vi "DT_Triangle Manager_Add Boundary.vi"(5 "point 2":i32, 6 "CCW? [T]":bool=TRUE, 7 "triangle 2":i32, 8 "point 1":i32, 9 "triangle 1":i32, 10 "apex point":i32, 11 "Triangles In":i32[][](array[numeric])) -> (0 "new triangle 2":i32, 1 "new triangle 1":i32, 2 "triangle":i32, 3 "Triangles Out":i32[][](array[numeric]))   [LabVIEW 2017, in "NI_AAL_Geometry.lvlib"]
uses:
  <vilib>/Analysis/NI_AAL_Geometry.lvlib
  <vilib>/Analysis/geometry.llb/DT_Triangle Manager_Get Global Point Index.vi
  <vilib>/Analysis/geometry.llb/DT_Triangle Manager_Get Oppo Point_in Ghost.vi
  <vilib>/Analysis/geometry.llb/DT_Triangle Manager_Get Oppo Point.vi
  <vilib>/Analysis/geometry.llb/DT_Triangle Manager_Default Ghost Index.vi
  <vilib>/Analysis/geometry.llb/DT_Triangle Manager_Get Ghost Point.vi
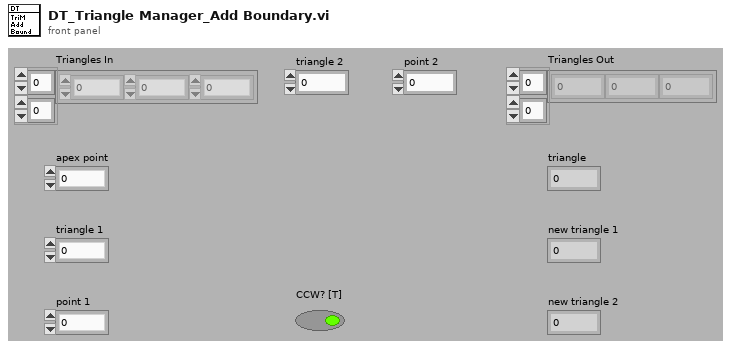
[diagram p1: front panel]
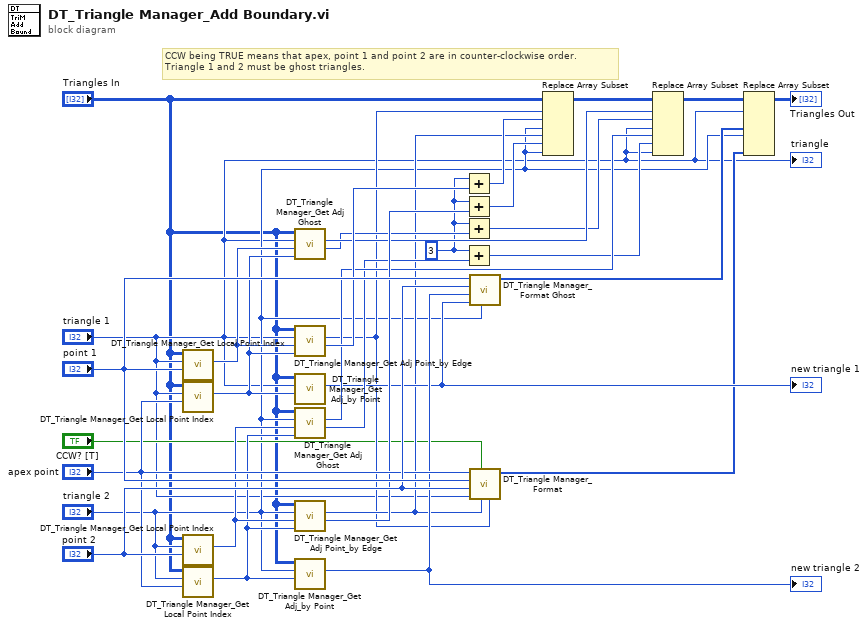
[diagram p0: block diagram]
diagram:
  w11 = 3 ("y")
  # "CCW being TRUE means that apex, point 1 and point 2 are in counter-clockwise order.\nTriangle 1 and 2 must be ghost triangles."
  n1 = call <vilib>:"DT_Triangle Manager_Get Local Point Index.vi"("global idx"="point 1", "triangle"="triangle 1", "Triangles"="Triangles In") -> ("local idx"=w23:i32)  [unwired: 8 out]
  n2 = call <vilib>:"DT_Triangle Manager_Get Local Point Index.vi"("global idx"="apex point", "triangle"="triangle 1", "Triangles"="Triangles In") -> ("local idx"=w22:i32)  [unwired: 8 out]
  n3 = call <vilib>:"DT_Triangle Manager_Get Local Point Index.vi"("global idx"="point 2", "triangle"="triangle 2", "Triangles"="Triangles In") -> ("local idx"=w18:i32)  [unwired: 8 out]
  n4 = call <vilib>:"DT_Triangle Manager_Get Local Point Index.vi"("global idx"="apex point", "triangle"="triangle 2", "Triangles"="Triangles In") -> ("local idx"=w17:i32)  [unwired: 8 out]
  n5 = call <vilib>:"DT_Triangle Manager_Get Adj Ghost.vi"("cur point idx"=w22, "cur base point idx"=w23, "cur triangle"="triangle 1", "Triangles In"="Triangles In") -> ("next base point idx"=w20:i32, "next triangle"=w21:i32)  [unwired: 6 out]
  n6 = call <vilib>:"DT_Triangle Manager_Get Adj Point_by Edge.vi"("point idx 2"=w22, "point idx 1"=w23, "triangle"="triangle 1", "Triangles In"="Triangles In") -> ("adj point idx"=w26:i32, "adj triangle"=w6:i32)  [unwired: 6 out]
  n7 = call <vilib>:"DT_Triangle Manager_Get Adj_by Point.vi"("point idx"=w22, "triangle"="triangle 1", "Triangles In"="Triangles In") -> ("adj triangle"=w9:i32)  [unwired: 8 out]
  "new triangle 1" <- w9
  n8 = call <vilib>:"DT_Triangle Manager_Get Adj Ghost.vi"("cur point idx"=w17, "cur base point idx"=w18, "cur triangle"="triangle 2", "Triangles In"="Triangles In") -> ("next base point idx"=w14:i32, "next triangle"=w16:i32)  [unwired: 6 out]
  n9 = call <vilib>:"DT_Triangle Manager_Get Adj Point_by Edge.vi"("point idx 2"=w17, "point idx 1"=w18, "triangle"="triangle 2", "Triangles In"="Triangles In") -> ("adj point idx"=w25:i32, "adj triangle"=w7:i32)  [unwired: 6 out]
  n10 = call <vilib>:"DT_Triangle Manager_Get Adj_by Point.vi"("point idx"=w17, "triangle"="triangle 2", "Triangles In"="Triangles In") -> ("adj triangle"=w10:i32)  [unwired: 8 out]
  "new triangle 2" <- w10
  n11 = Add(x=w11, y=w26) -> (x+y=w28:i32)
  n12 = Add(x=w11, y=w25) -> (x+y=w27:i32)
  n13 = Add(x=w11, y=w20) -> (x+y=w19:i32)
  n14 = Add(x=w11, y=w14) -> (x+y=w15:i32)
  n15 = call <vilib>:"DT_Triangle Manager_Format Ghost.vi"("triangle"="triangle 2", "p 2 triangle"=w9, "p 1 triangle"=w10, "p 2"="point 2", "p 1"="point 1") -> ("Triangle"=w8:i32[])  [unwired: 6 out]
  n16 = call <vilib>:"DT_Triangle Manager_Format.vi"("p 3 triangle"=w6, "p 2 triangle"=w7, "CCW? [T]"="CCW? [T]", "p 1 triangle"="triangle 1", "p 3"="point 2", "p 2"="point 1", "p 1"="apex point") -> ("Triangle"=w5:i32[])  [unwired: 4 out]
  n17 = Replace Array Subset(array="Triangles In", new element #1="triangle 2", index (row) #1=w6, index (col) #1=w28, new element #2="triangle 2", index (row) #2=w7, index (col) #2=w27) -> (w24:i32[][])
  n18 = Replace Array Subset(array=w24, new element #1="triangle 1", index (row) #1=w21, index (col) #1=w19, new element #2="triangle 1", index (row) #2=w16, index (col) #2=w15) -> (w13:i32[][])
  n19 = Replace Array Subset(array=w13, new element #1=w8, index (row) #1="triangle 1", new element #2=w5, index (row) #2="triangle 2") -> (→"Triangles Out":i32[][])  [unwired: 2 in]
  "triangle" <- "triangle 1"
